vi "Shutdown.vi"(8 "error in (no error)":errorcluster, 11 "Temp01 in":refnum<class "TELLC_Temp01.lvclass">) -> (0 "error out":errorcluster, 3 "Temp01 out":refnum<class "TELLC_Temp01.lvclass">)   [LabVIEW 2017, in "TELLC_Temp01.lvclass"]
doc: "Developed by Kevin Thompson\nkevin@thompsonengineering.net\n\nCopyright 2018\nThompson Engineering, LLC"
uses:
  TELLC_Temp01.lvclass
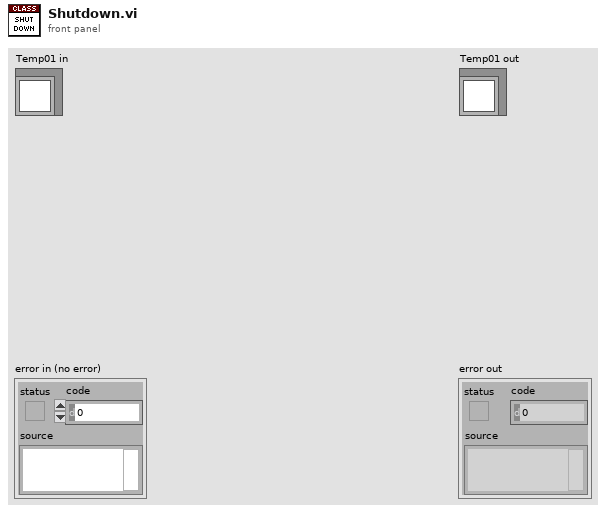
[diagram p1: front panel]
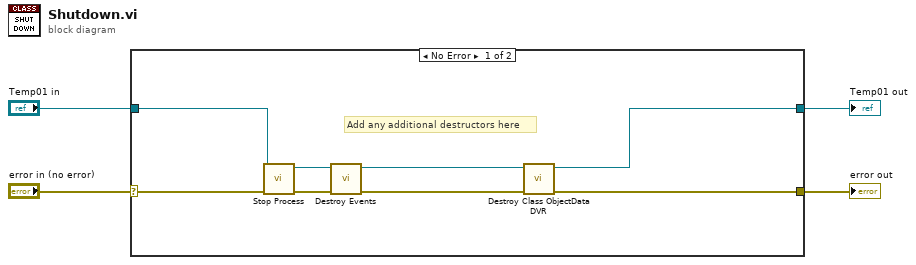
[diagram p0: block diagram]
diagram:
  n1 = case shown="No Error" "error in (no error)" {
    selector: "error in (no error)" -> [w12 w14]
    tunnel: [w7 w14] -> w3
    tunnel: [w5 w13] -> w1
    tunnel: "Temp01 in" -> [w10 w13]
    frame No Error {
      # "Add any additional destructors here"
      n2 = call "Stop Process.vi"("error in (no error)"=w12, "Temp01 in"=w10) -> ("error out"=w11:errorcluster, "Temp01 out"=w9:refnum<class "TELLC_Temp01.lvclass">)  [unwired: 8 in]
      n3 = call "Destroy Events.vi"("error in (no error)"=w11, "Temp01 in"=w9) -> ("error out"=w8:errorcluster, "Temp01 out"=w6:refnum<class "TELLC_Temp01.lvclass">)  [unwired: 8 in]
      n4 = call "Destroy Class ObjectData DVR.vi"("error in (no error)"=w8, "Temp01 in"=w6) -> ("error out"=w7:errorcluster, "Temp01 out"=w5:refnum<class "TELLC_Temp01.lvclass">)  [unwired: 8 in]
    }
    frame Error {
    }
  }
  "error out" <- w3
  "Temp01 out" <- w1
